vi "Get Simulation Enabled For Operator Mode.vi"(11 "error in (no error)":errorcluster) -> (4 "Use Simulated Instrument?":bool, 6 "Use Operator Mode?":bool, 15 "error out":errorcluster)   [LabVIEW 2023, in "RFCalAndFixtureCharact.Common.lvlib"]
uses:
  RFCalAndFixtureCharact.Common.lvlib
  Data Cache/Settings Dictionary/Setting Keys.vi
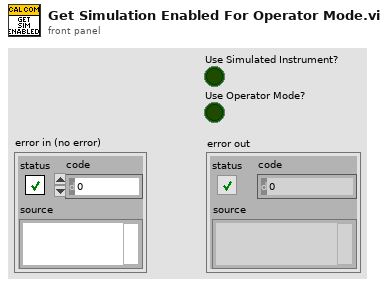
[diagram p1: front panel]
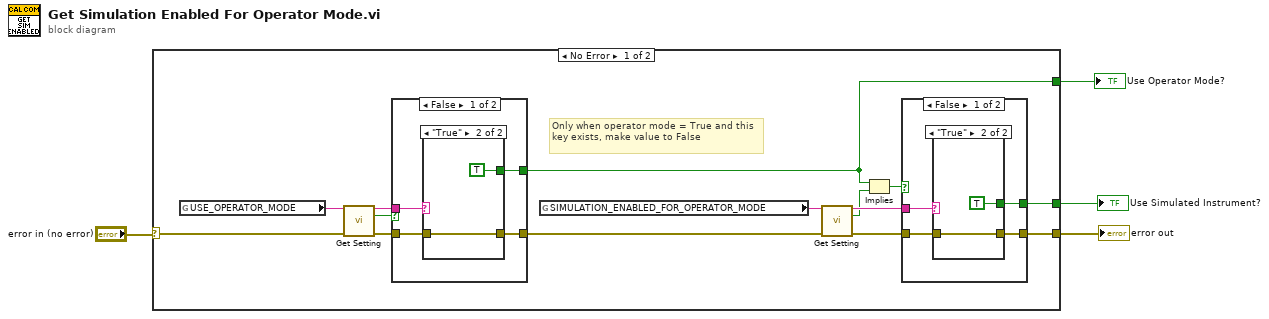
[diagram p0: block diagram]
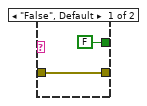
[diagram p2: hidden frame]
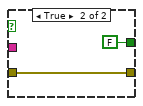
[diagram p3: hidden frame]
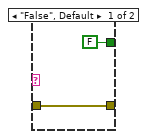
[diagram p4: hidden frame]
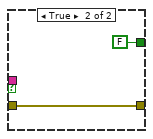
[diagram p5: hidden frame]
diagram:
  n1 = case shown="No Error" "error in (no error)" {
    selector: "error in (no error)" -> [w11 w39]
    tunnel: [w18 w39] -> w3
    tunnel: [w17 _] -> w2
    tunnel: [w6 _] -> w1
    frame No Error {
      # "Only when operator mode = True and this key exists, make value to False"
      n2 = global read "Setting Keys.vi" "USE_OPERATOR_MODE"() -> (w8:string)
      n3 = call "Get Setting.vi"("Setting name"=w8, "error in (no error)"=w11) -> ("Setting value out"=w7:string, "Setting empty or not found?"=w9:bool, "error out"=w10:errorcluster)  [unwired: 11 in]
      n4 = case shown="False" w9 {
        tunnel: [w31 w38] -> w5
        tunnel: w10 -> [w30 w38]
        tunnel: w7 -> [w32 _]
        tunnel: [w29 FALSE] -> w6
        frame False {
          n5 = case shown="\"True\"" w32 {
            tunnel: [w34 w36] -> w31
            tunnel: w30 -> [w34 w36]
            tunnel: [FALSE TRUE] -> w29
            frame "False", Default {
            }
            frame "True" {
            }
          }
        }
        frame True {
        }
      }
      n6 = global read "Setting Keys.vi" "SIMULATION_ENABLED_FOR_OPERATOR_MODE"() -> (w16:string)
      n7 = call "Get Setting.vi"("Setting name"=w16, "error in (no error)"=w5) -> ("Setting value out"=w14:string, "Setting empty or not found?"=w12:bool, "error out"=w15:errorcluster)  [unwired: 11 in]
      n8 = Implies(1:w12, 2:w6) -> (0:w13:bool)
      n9 = case shown="False" w13 {
        tunnel: [w21 w28] -> w18
        tunnel: w15 -> [w20 w28]
        tunnel: w14 -> [w22 _]
        tunnel: [w19 FALSE] -> w17
        frame False {
          n10 = case shown="\"True\"" w22 {
            tunnel: [w24 w26] -> w21
            tunnel: w20 -> [w24 w26]
            tunnel: [FALSE TRUE] -> w19
            frame "False", Default {
            }
            frame "True" {
            }
          }
        }
        frame True {
        }
      }
    }
    frame Error {
    }
  }
  "error out" <- w3
  "Use Simulated Instrument?" <- w2
  "Use Operator Mode?" <- w1
